vi "loop-for.vi"() -> ()   [LabVIEW 2020, in "Library 1.lvlib"]
uses:
  Libs/Library 1.lvlib
panel:
  in  "N VALUE":dbl
  out "Slide 2":dbl(slide) scale=0.0..100.0
  out "1 VALUE":i32
  in  "ARRAY 2 -1":dbl
  in  "ARRAY 1-1":dbl
  in  "ARRA 2-2":dbl
  in  "ARRAY 1 -0":dbl
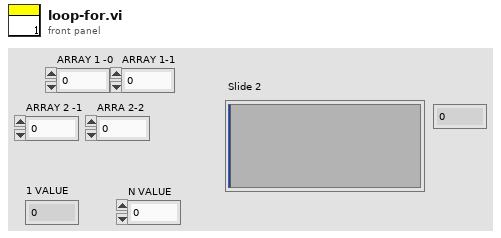
[diagram p1: front panel]
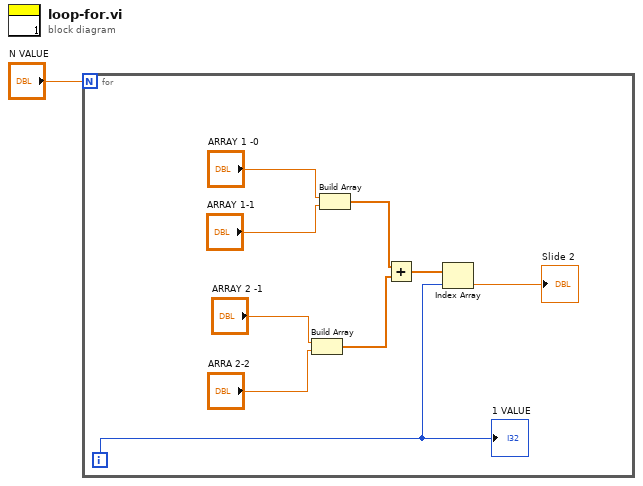
[diagram p0: block diagram]
diagram:
  n1 = for {
    N: "N VALUE" -> [_]
    i -> [w3]
    n2 = Build Array("ARRAY 2 -1", "ARRA 2-2") -> (w5:dbl[])
    n3 = Build Array("ARRAY 1 -0", "ARRAY 1-1") -> (w6:dbl[])
    n4 = Add(x=w6, y=w5) -> (x+y=w4:dbl[])
    n5 = Index Array(array=w4, index=w3) -> (element=→"Slide 2":dbl)
    "1 VALUE" <- w3
  }
